vi "Serial Monitor.vi"() -> ()   [LabVIEW 2020]
uses:
  <vilib>/Instr/_visa.llb/VISA Configure Serial Port (Instr).vi
panel:
  in  "stop":bool
  in  "baud rate (9600)":u32=1000000
  in  "Array":u32[](array[numeric])=[1000, 1000, 1000, 1000]
  in  "Set_vel":bool
  in  "Média":i32=1
  out "Waveform Chart":T1(graph)
  in  "VISA resource name":refnum<visa-resource-name>
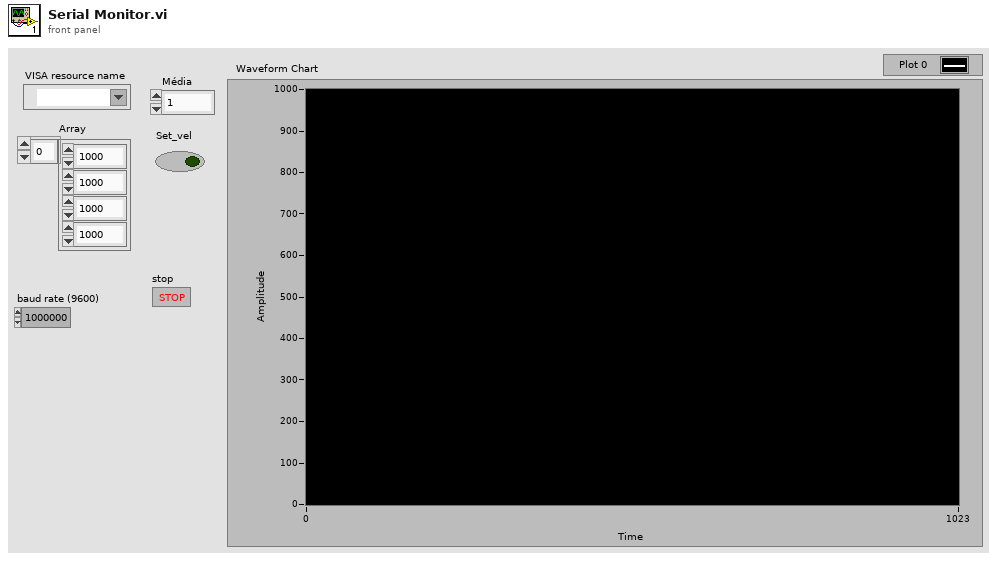
[diagram p1: front panel]
types:
  T1 = cluster{"[0]":dbl, "[1]":dbl, "[2]":dbl, "[3]":dbl, "[4]":dbl, "[5]":dbl, "[6]":dbl, "[7]":dbl, "[8]":dbl}
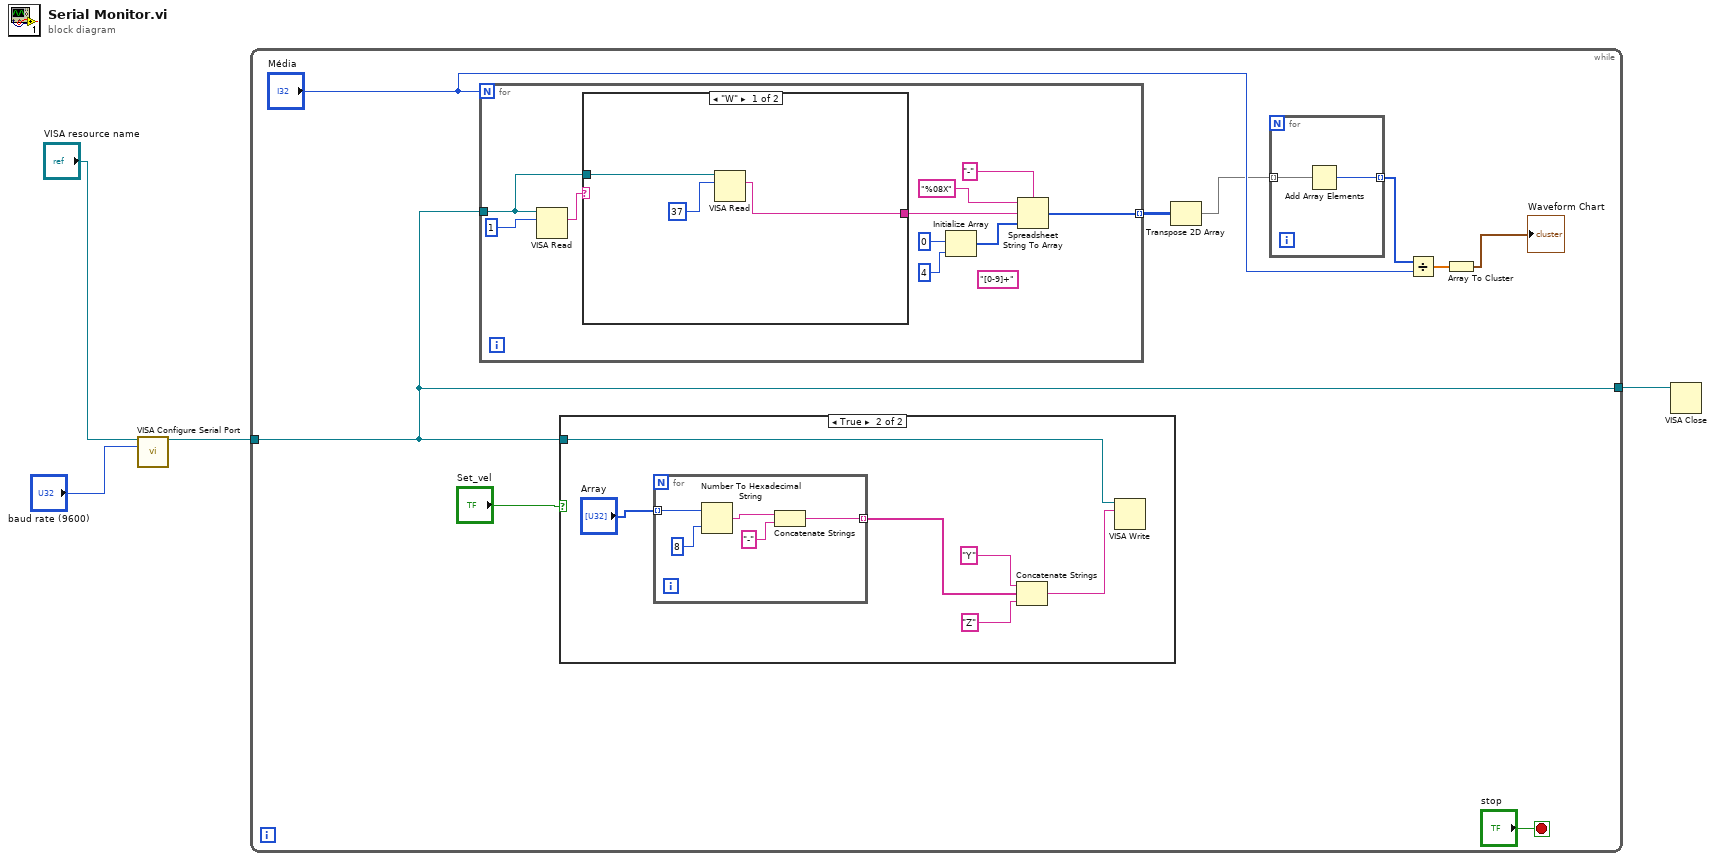
[diagram p0: block diagram]
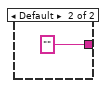
[diagram p3: hidden frame]
diagram:
  n1 = call-poly "VISA Configure Serial Port"("VISA resource name"="VISA resource name", "baud rate (9600)"="baud rate (9600)") -> ("VISA resource name out"=w4:refnum<visa-resource-name>)  [unwired: 12 in, 1 out]
  n2 = while {
    tunnel: w4 -> [w5]
    tunnel: [w5] -> w1
    stop <- "stop" stop-if-true
    n3 = for {
      N: "Média" -> [_]
      tunnel: w5 -> [w34]
      tunnel: [w27] -> w10 mode=indexing
      (unwired) "[0-9]+" ("regular expression")
      n4 = VISA Read(VISA resource name=w34, byte count=u32 1) -> (read buffer=w35:string)  [unwired: 1 in, 3 out]
      n5 = case shown="\"W\"" w35 {
        tunnel: w34 -> [w39 _]
        tunnel: [w38 "" ("read buffer")] -> w33
        frame "W" {
          n6 = VISA Read(VISA resource name=w39, byte count=u32 37) -> (read buffer=w38:string)  [unwired: 1 in, 3 out]
        }
        frame Default {
        }
      }
      n7 = Initialize Array(0, 4 ("dimension size")) -> (w28:i32[])
      n8 = Spreadsheet String To Array(delimiter (Tab)="-", format string="%08X", spreadsheet string=w33, array type (2D Dbl)=w28) -> (array=w27:i32[])
    }
    n9 = case shown="True" "Set_vel" {
      tunnel: w5 -> [_ w21]
      frame False {
      }
      frame True {
        n10 = for {
          tunnel: "Array" -> [w26] mode=indexing
          tunnel: [w23] -> w19 mode=indexing
          n11 = Number To Hexadecimal String(1:i16 8 ("width (-)"), 2:w26) -> (0:w25:string)
          n12 = Concatenate Strings(w25, "-" ("string")) -> (w23:string)
        }
        n13 = Concatenate Strings("Y", w19, "Z") -> (w20:string)
        n14 = VISA Write(VISA resource name=w21, write buffer=w20) -> ()  [unwired: 1 in, 3 out]
      }
    }
    n15 = Transpose 2D Array(2D array=w10) -> (transposed array=w9:i32[][])
    n16 = for {
      tunnel: w9 -> [w15] mode=indexing
      tunnel: [w14] -> w11 mode=indexing
      n17 = Add Array Elements(numeric array=w15) -> (sum=w14:i32)
    }
    n18 = Divide(x=w11, y="Média") -> (x/y=w8:dbl[])
    n19 = Array To Cluster(array=w8) -> (cluster=→"Waveform Chart":T1)
  }
  n20 = VISA Close(VISA resource name=w1) -> ()  [unwired: 1 in, 1 out]
